vi "PerpendicularPointA_DestTarget.vi"(6 "Ball (x,y)":dbl[](array[numeric]), 7 "Raio":dbl, 8 "error in (no error)":errorcluster, 9 "Robot - Ball":dbl[](array[numeric]) format="%0.2f", 10 "Ball - Target":dbl[](array[numeric]) format="%0.2f", 11 "KickToSkill in":refnum<class "KickToSkill.lvclass">) -> (0 "error out":errorcluster, 2 "Ponto A":dbl[](array[numeric]), 3 "KickToSkill out":refnum<class "KickToSkill.lvclass">)   [LabVIEW 2021, in "KickToSkill.lvclass"]
uses:
  KickToSkill.lvclass
  <vilib>/Analysis/coordinate.llb/2D Cartesian Coordinate Rotation (Scalar).vi
  <vilib>/Analysis/NI_AALPro.lvlib
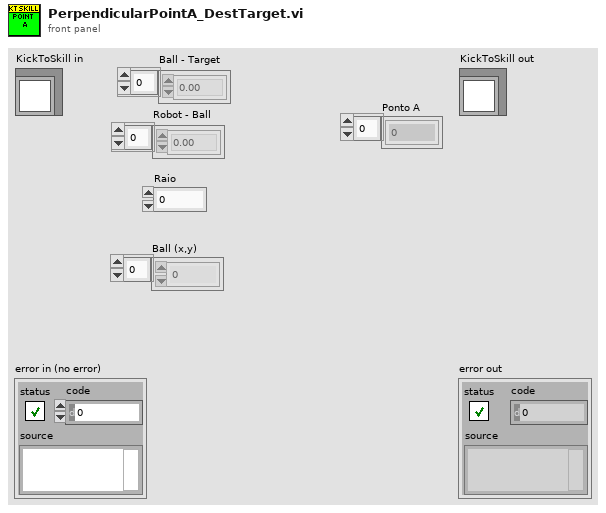
[diagram p1: front panel]
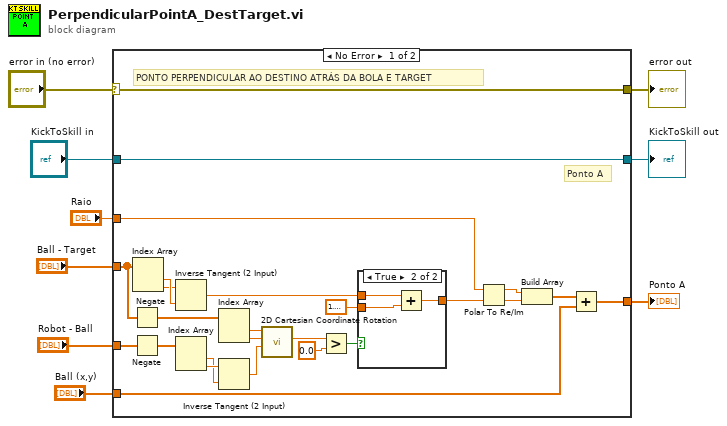
[diagram p0: block diagram]
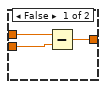
[diagram p2: hidden frame]
diagram:
  n1 = case shown="No Error" "error in (no error)" {
    selector: "error in (no error)" -> [w34 w42]
    tunnel: [w34 w42] -> w8
    tunnel: [w12 w41] -> w7
    tunnel: "KickToSkill in" -> [w12 w41]
    tunnel: [w15 _] -> w6
    tunnel: "Ball (x,y)" -> [w14 _]
    tunnel: "Raio" -> [w13 _]
    tunnel: "Ball - Target" -> [w11 _]
    tunnel: "Robot - Ball" -> [w10 _]
    frame No Error {
      # "PONTO PERPENDICULAR AO DESTINO ATRÁS DA BOLA E TARGET"
      # "Ponto A"
      n2 = Negate(x=w11) -> (-x=w21:dbl[])
      n3 = Negate(x=w10) -> (-x=w18:dbl[])
      n4 = Index Array(array=w11) -> (element #1=w33:dbl, element #2=w32:dbl)  [unwired: 2 in]
      n5 = Inverse Tangent (2 Input)(1:w33, 2:w32) -> (0:w31:dbl)
      n6 = Index Array(array=w18) -> (element #1=w19:dbl, element #2=w20:dbl)  [unwired: 2 in]
      n7 = Index Array(array=w21) -> (element #1=w22:dbl, element #2=w23:dbl)  [unwired: 2 in]
      n8 = Inverse Tangent (2 Input)(1:w19, 2:w20) -> (0:w17:dbl)
      n9 = call-poly <vilib>:"2D Cartesian Coordinate Rotation.vi"("theta"=w17, "y"=w23, "x"=w22) -> ("y out"=w16:dbl)  [unwired: 6 in, 2 out]
      n10 = Greater?(x=w16, y=0.0) -> (0:w24:bool)
      n11 = case shown="True" w24 {
        tunnel: w31 -> [w36 w40]
        tunnel: 1.5707963267948966 -> [w37 w39]
        tunnel: [w35 w38] -> w28
        frame False {
          n12 = Subtract(x=w36, y=w37) -> (x-y=w35:dbl)
        }
        frame True {
          n13 = Add(x=w40, y=w39) -> (x+y=w38:dbl)
        }
      }
      n14 = Polar To Re/Im(2:w28, 3:w13) -> (0:w26:dbl, 1:w27:dbl)
      n15 = Build Array(w27, w26) -> (w25:dbl[])
      n16 = Add(x=w25, y=w14) -> (x+y=w15:dbl[])
    }
    frame Error {
    }
  }
  "error out" <- w8
  "KickToSkill out" <- w7
  "Ponto A" <- w6
